vi "List Basic Types.vi"() -> (1 "Short Class Names":string[](array[string]), 2 "Long Class Names":string[](array[string]), 3 "Basic Types":refnum<class "Tree Data.lvclass">[](array[class]))   [LabVIEW 2017, in "Tree API.lvlib" / "Tree.lvclass"]
doc: "Return a list of all basic Tree Data types used by Tree API"
uses:
  Tree.lvclass
  Data Types/Bool Array/1D Bool.lvclass
  Data Types/Bool/Bool.lvclass
  Data Types/Flt Array/1D Flt.lvclass
  Data Types/Float/Flt.lvclass
  Data Types/Int Array/1D Int.lvclass
  Data Types/Int/Int.lvclass
  Data Types/Path Array/1D Path.lvclass
  Data Types/Path/Path.lvclass
  Data Types/String Array/1D String.lvclass
  Data Types/String/String.lvclass
  Data Types/2D Bool/2D Bool.lvclass
  Data Types/2D Int/2D Int.lvclass
  Data Types/2D Flt/2D Flt.lvclass
  Data Types/2D Path/2D Path.lvclass
  Data Types/2D String/2D String.lvclass
  Tree Data/Tree Data.lvclass
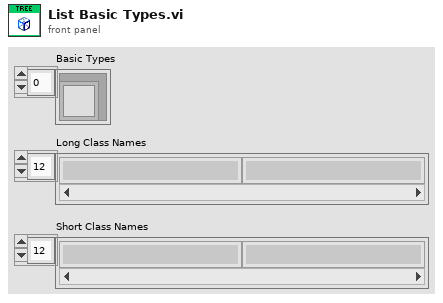
[diagram p1: front panel]
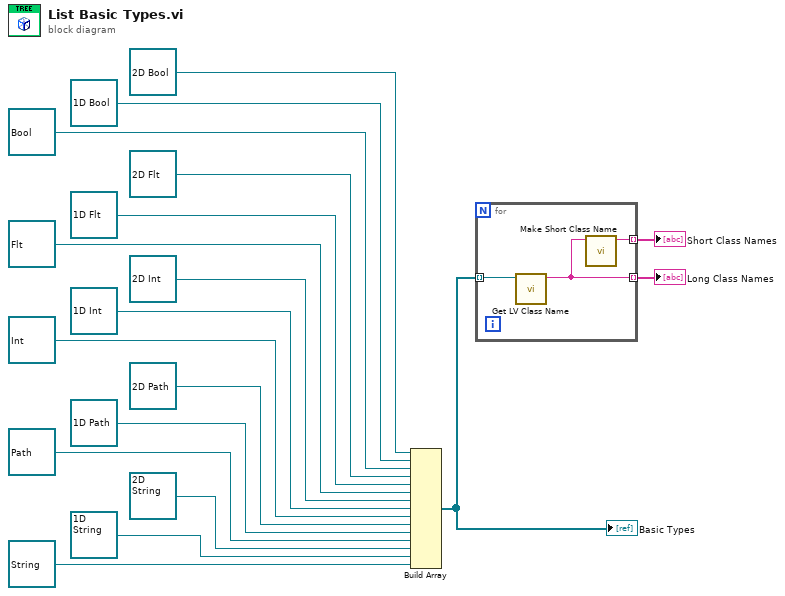
[diagram p0: block diagram]
diagram:
  n1 = Build Array(refnum<class "2D Bool.lvclass"> refnum ("Tree API.lvlib:2D Bool.lvclass"), refnum<class "1D Bool.lvclass"> refnum ("Bool Array.lvclass"), refnum<class "Bool.lvclass"> refnum ("Bool.lvclass"), refnum<class "2D Flt.lvclass"> refnum ("Tree API.lvlib:2D Flt.lvclass"), refnum<class "1D Flt.lvclass"> refnum ("Flt Array.lvclass"), refnum<class "Flt.lvclass"> refnum ("Flt.lvclass"), refnum<class "2D Int.lvclass"> refnum ("Tree API.lvlib:2D Int.lvclass"), refnum<class "1D Int.lvclass"> refnum ("Int Array.lvclass"), refnum<class "Int.lvclass"> refnum ("Int.lvclass"), refnum<class "2D Path.lvclass"> refnum ("Tree API.lvlib:2D Path.lvclass"), refnum<class "1D Path.lvclass"> refnum ("Path Array.lvclass"), refnum<class "Path.lvclass"> refnum ("Path.lvclass"), refnum<class "2D String.lvclass"> refnum ("Tree API.lvlib:2D String.lvclass"), refnum<class "1D String.lvclass"> refnum ("String Array.lvclass"), refnum<class "String.lvclass"> refnum ("String.lvclass")) -> (w7:refnum<class "Tree Data.lvclass">[])
  "Basic Types" <- w7
  n2 = for {
    tunnel: w7 -> [w21] mode=indexing
    tunnel: [w20] -> w8 mode=indexing
    tunnel: [w19] -> w6 mode=indexing
    n3 = call <vilib>:"Get LV Class Name.vi"("object"=w21) -> ("class name"=w20:string)  [unwired: 9 in, 1 out]
    n4 = call "Make Short Class Name.vi"("Class Name"=w20) -> ("Shortened Class Name"=w19:string)  [unwired: 10 in]
  }
  "Long Class Names" <- w8
  "Short Class Names" <- w6
